vi "Get Debug.vi"(8 "error in (no error)":errorcluster, 11 "VISA resource name":refnum<visa-resource-name>) -> (0 "error out":errorcluster, 2 "output":string, 3 "VISA resource name out":refnum<visa-resource-name>)   [LabVIEW 2024, in "Detector SCPI.lvlib"]
doc: "Returns string with debug information from SCPI parser"
uses:
  <instrlib>/Detector SCPI/Detector SCPI.lvlib
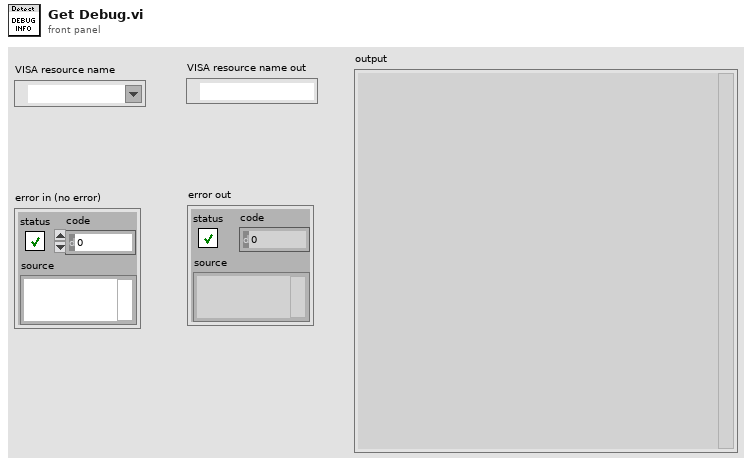
[diagram p1: front panel]
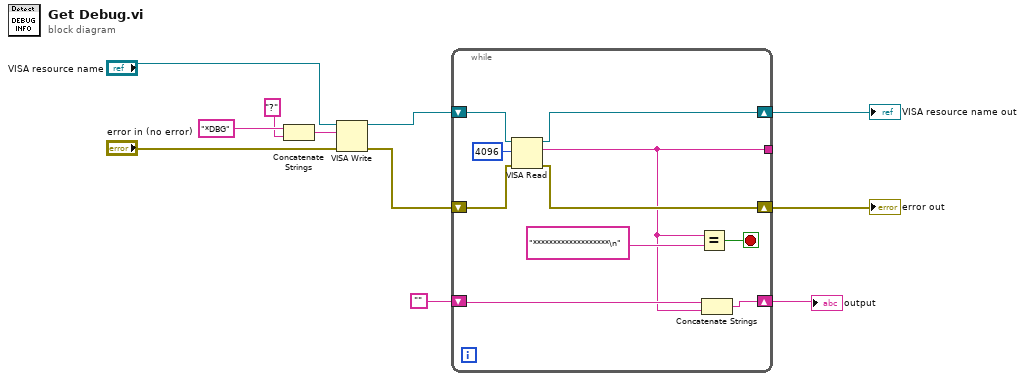
[diagram p0: block diagram]
diagram:
  n1 = Concatenate Strings("*DBG" ("command"), "?" ("command")) -> (w8:string)
  n2 = VISA Write(VISA resource name="VISA resource name", write buffer=w8, error in (no error)="error in (no error)") -> (VISA resource name out=w3:refnum<visa-resource-name>, error out=w9:errorcluster)  [unwired: 1 out]
  n3 = while {
    tunnel: [w12] -> _
    shift-right: [w18] -> w4
    shift-left: w9 -> [w21]
    shift-right: [w20] -> w5
    shift-left: w3 -> [w17]
    shift-right: [w14] -> w2
    shift-left: "" -> [w13]
    stop <- w16 stop-if-true
    n4 = VISA Read(VISA resource name=w17, byte count=u32 4096, error in (no error)=w21) -> (VISA resource name out=w20:refnum<visa-resource-name>, read buffer=w12:string, error out=w18:errorcluster)  [unwired: 1 out]
    n5 = Equal?(x=w12, y="*******************\n") -> (x = y?=w16:bool)
    n6 = Concatenate Strings(w13, w12) -> (w14:string)
  }
  "VISA resource name out" <- w5
  "error out" <- w4
  "output" <- w2
